vi "io_read_long_data.vi"(4 "Simulation read buffer (\"Simulation\")":string="Simulation", 6 "Block Logging (F)":bool, 8 "error in":errorcluster, 10 "Max chunk read bytes count (65536)":u32=65536, 11 "VISA resource name":refnum<visa-resource-name>) -> (0 "error out":errorcluster, 1 "return count":u32, 2 "read buffer":string, 3 "VISA resource name out":refnum<visa-resource-name>)   [LabVIEW 2014, in "rszvl_rsidr_core.lvlib"]
uses:
  rszvl_rsidr_core.lvlib
  type_Error_Codes.ctl
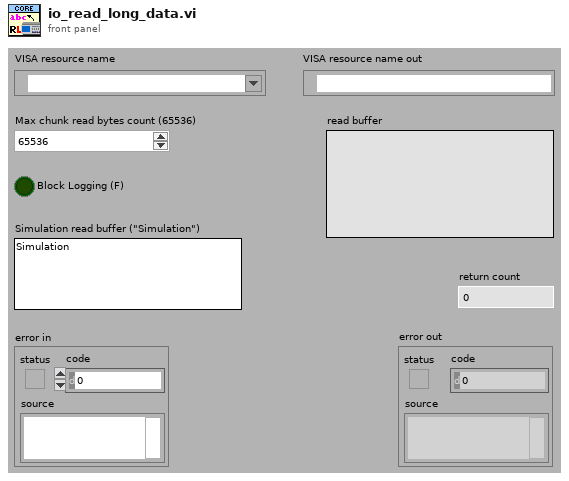
[diagram p1: front panel]
types:
  T1 = typedef "rszvl_rsidr_core.lvlib/type_Error_Codes.ctl" = enum16{"No_error", "VISA_err_ResourceNotFound", "VISA_err_Timeout", "VISA_warn_MoreDataAvailable", "RS_err_MissingCallback", "RS_err_InvalidAttribute", "RS_err_InvalidValue", "RS_err_UnknownResource", "RS_err_AlreadyInitialized", "RS_err_InstrumentStatus", "RS_err_BadRepCapName", "RS_err_TypesMismatch", "RS_err_ValueNotSupported", "RS_err_InvalidRngTable", "RS_err_IDqueryFail", "RS_err_UnexpResponse", "VISA_warn_ConfigNotLoaded", "RS_err_AttributeNotReadable", "RS_err_AttributeNotWritable", "RS_err_InstrumentType", "RS_err_InstrumentOption", "VISA_err_InvalidSize", "RS_err_ReliabilityIndicator", "VISA_warn_UnknownStatus", "VISA_warn_TermCharRead", "VISA_err_IO_error"}
  T2 = typedef "rszvl_rsidr_core.lvlib/type_Session_Data.ctl" = cluster{"Instr type":string, "Instr type for err. msg.":string, "Installed Options":string[], "OPC Timeout":i32, "Query Instrument Status":bool, "Check Range":bool, "Check Options":bool, "Add LF to Write":bool, "Simulate":bool, "Logging":bool, "Logging params":variant, "Interface Type":enum16{"Unknown", "GPIB", "VXI", "GPIB_VXI", "ASRL", "PXI", "TCPIP", "USB", "SOCKET"}, "Fast Sweep":i32, "AdditionalFlags":i32, "WaitBeforeWrite":i32, "WaitBeforeRead":i32, "BinDataChunkSize":i64}
  T3 = enum16{"Unknown", "GPIB", "VXI", "GPIB_VXI", "ASRL", "PXI", "TCPIP", "USB", "SOCKET"}
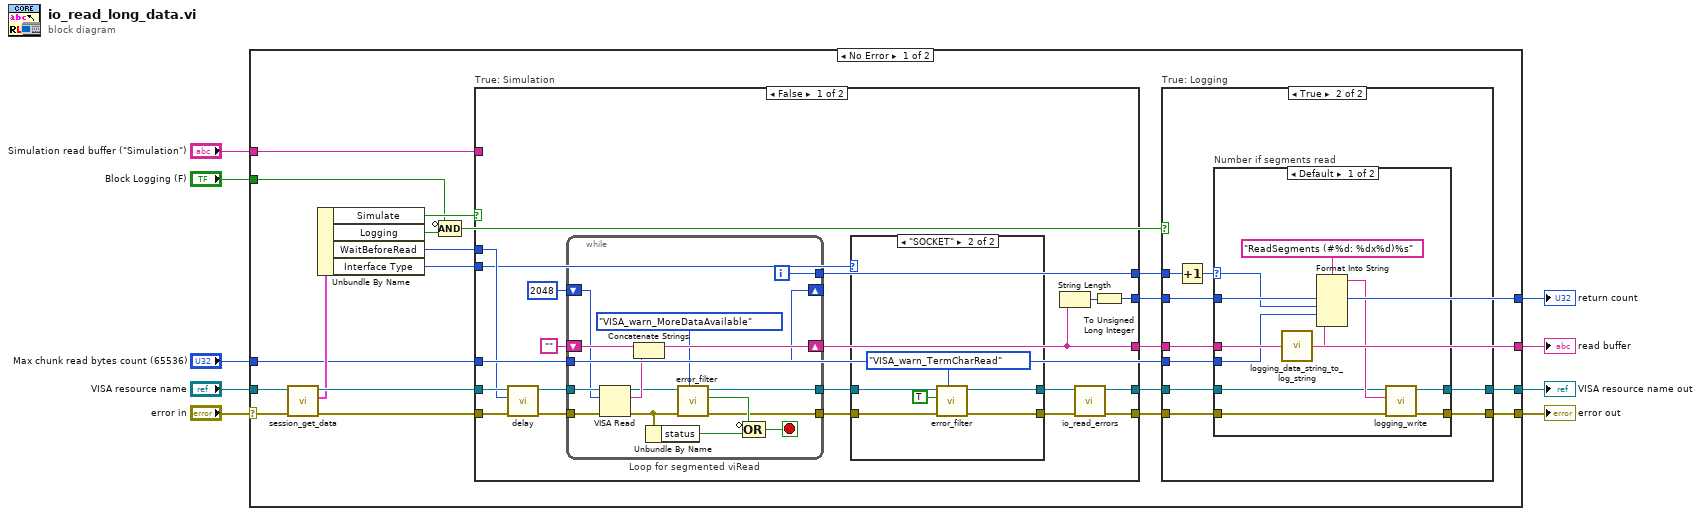
[diagram p0: block diagram]
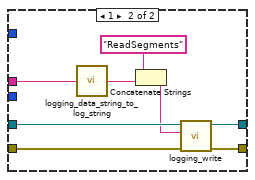
[diagram p3: hidden frame]
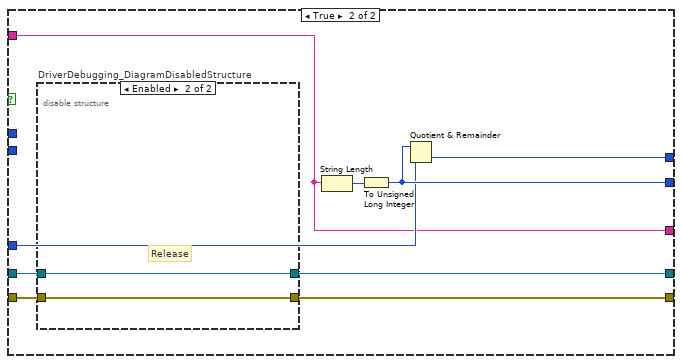
[diagram p5: hidden frame]
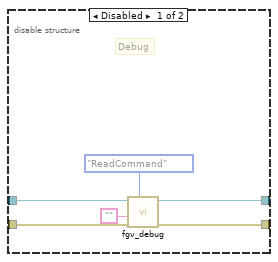
[diagram p6: hidden frame]
diagram:
  n1 = case shown="No Error" "error in" {
    selector: "error in" -> [w29 w121]
    tunnel: [w20 w121] -> w4
    tunnel: "Max chunk read bytes count (65536)" -> [w15 _]
    tunnel: [w16 _] -> w8
    tunnel: "VISA resource name" -> [w28 w120]
    tunnel: [w17 _] -> w5
    tunnel: [w19 w120] -> w3
    tunnel: "Simulation read buffer (\"Simulation\")" -> [w11 _]
    tunnel: "Block Logging (F)" -> [w10 _]
    frame No Error {
      n2 = call "session_get_data.vi"("error in"=w29, "VISA resource name"=w28) -> ("error out"=w27:errorcluster, "Session User Data out"=w25:T2, "VISA resource name out"=w26:refnum<visa-resource-name>)  [unwired: 7 in]
      n3 = Unbundle By Name(w25) -> ("Simulate"=w24:bool, "Logging"=w23:bool, "WaitBeforeRead"=w13:i32, "Interface Type"=w12:T3)
      n4 = Compound Arithmetic op=AND(invert w10, w23) -> (w14:bool)
      n5 = case "True: Simulation" shown="False" w24 {
        tunnel: [w73 w105] -> w22
        tunnel: [w76 w103] -> w16
        tunnel: [w78 w109] -> w17
        tunnel: w27 -> [w71 w107]
        tunnel: w26 -> [w70 w106]
        tunnel: [w72 w104] -> w21
        tunnel: w15 -> [w60 w108]
        tunnel: [w74 w110] -> w18
        tunnel: w13 -> [w67 _]
        tunnel: w12 -> [w64 _]
        tunnel: w11 -> [_ w103]
        frame False {
          n6 = call "delay.vi"("error in"=w71, "Milliseconds to wait"=w67, "VISA resource name"=w70) -> ("error out"=w69:errorcluster, "VISA resource name out"=w68:refnum<visa-resource-name>)  [unwired: 7 in]
          n7 = while "Loop for segmented viRead" {
            shift-left: "" ("Empty String Constant") -> [w101]
            shift-right: [w99] -> w76
            tunnel: w68 -> [w102]
            tunnel: w69 -> [w100]
            tunnel: [w92] -> w66
            tunnel: [w89] -> w63
            tunnel: [w91] -> w74
            shift-right: [w87] -> _
            shift-left: u32 2048 ("Max chunk read bytes count (65536)") -> [w88]
            tunnel: w60 -> [w87]
            i -> [w91]
            stop <- w96 stop-if-true
            n8 = VISA Read(VISA resource name=w102, byte count=w88, error in (no error)=w100) -> (VISA resource name out=w90:refnum<visa-resource-name>, read buffer=w93:string, error out=w98:errorcluster)  [unwired: 1 out]
            n9 = Concatenate Strings(w101, w93) -> (w99:string)
            n10 = Unbundle By Name(w98) -> ("status"=w97:bool)
            n11 = call "error_filter.vi"("Error Enum in"=type_Error_Codes."VISA_warn_MoreDataAvailable" ("Code to detect"), "error in"=w98, "VISA resource name"=w90) -> ("error out"=w92:errorcluster, "Code Detected"=w94:bool, "VISA resource name out"=w89:refnum<visa-resource-name>)  [unwired: 6 in]
            n12 = Compound Arithmetic op=OR(invert w94, w97) -> (w96:bool)
          }
          n13 = case shown="\"SOCKET\"" w64 {
            tunnel: w66 -> [w80 w86]
            tunnel: [w80 w84] -> w65
            tunnel: w63 -> [w79 w82]
            tunnel: [w79 w81] -> w62
            frame Default {
            }
            frame "SOCKET" {
              n14 = call "error_filter.vi"("Error Enum in"=type_Error_Codes."VISA_warn_TermCharRead" ("Code to detect"), "error in"=w86, "Clear detected code (F)"=TRUE, "VISA resource name"=w82) -> ("error out"=w84:errorcluster, "VISA resource name out"=w81:refnum<visa-resource-name>)  [unwired: 5 in, 1 out]
            }
          }
          n15 = String Length(string=w76) -> (length=w75:i32)
          n16 = call "io_read_errors.vi"("error in"=w65, "VISA resource name"=w62) -> ("error out"=w73:errorcluster, "VISA resource name out"=w72:refnum<visa-resource-name>)  [unwired: 8 in]
          n17 = To Unsigned Long Integer(number=w75) -> (unsigned 32bit integer=w78:u32)
        }
        frame True {
          n18 = disable-structure "DriverDebugging_DiagramDisabledStructure" shown="Enabled" {
            disable-tunnel: w107 -> [w116 w118]
            disable-tunnel: [w114 w118] -> w105
            disable-tunnel: w106 -> [w115 w119]
            disable-tunnel: [w113 w119] -> w104
            frame Disabled {
              # "Debug"
              n19 = call "fgv_debug.vi"("Operation"=enum16{"Reset", "ReadCommand", "SetCommand"}."ReadCommand", "error in"=w116, "Command in"="" ("Empty String Constant"), "VISA resource name"=w115) -> ("error out"=w114:errorcluster, "VISA resource name out"=w113:refnum<visa-resource-name>)  [unwired: 6 in]
            }
            frame Enabled {
              # "Release"
            }
          }
          n20 = String Length(string=w103) -> (length=w111:i32)
          n21 = To Unsigned Long Integer(number=w111) -> (unsigned 32bit integer=w109:u32)
          n22 = Quotient & Remainder(x=w109, y=w108) -> (floor(x/y)=w110:u32)  [unwired: 1 out]
        }
      }
      n23 = case "True: Logging" shown="True" w14 {
        tunnel: w21 -> [w30 w34]
        tunnel: w22 -> [w31 w35]
        tunnel: [w31 w33] -> w20
        tunnel: [w30 w32] -> w19
        tunnel: w18 -> [_ w39]
        tunnel: w16 -> [_ w40]
        tunnel: w17 -> [_ w37]
        tunnel: w15 -> [_ w36]
        frame False {
        }
        frame True {
          n24 = Increment(x=w39) -> (x+1=w38:u32)
          n25 = case "Number if segments read" shown="Default" w38 {
            selector: w38 -> [w43 _]
            tunnel: w35 -> [w49 w59]
            tunnel: w34 -> [w48 w58]
            tunnel: [w47 w57] -> w33
            tunnel: [w46 w56] -> w32
            tunnel: w40 -> [w50 w55]
            tunnel: w37 -> [w44 _]
            tunnel: w36 -> [w42 _]
            frame Default {
              n26 = call "logging_data_string_to_log_string.vi"("Raw string to log"=w50) -> ("Result log string"=w41:string)  [unwired: 4 in]
              n27 = Format Into String(format string="ReadSegments (#%d: %dx%d)%s", w44, w43, w42, w41) -> (resulting string=w51:string)  [unwired: 2 in, 1 out]
              n28 = call "logging_write.vi"("error in"=w49, "String to write"=w51, "VISA resource name"=w48) -> ("error out"=w47:errorcluster, "VISA resource name out"=w46:refnum<visa-resource-name>)  [unwired: 7 in]
            }
            frame 1 {
              n29 = call "logging_data_string_to_log_string.vi"("Raw string to log"=w55) -> ("Result log string"=w54:string)  [unwired: 4 in]
              n30 = Concatenate Strings("ReadSegments" ("format string"), w54) -> (w52:string)
              n31 = call "logging_write.vi"("error in"=w59, "String to write"=w52, "VISA resource name"=w58) -> ("error out"=w57:errorcluster, "VISA resource name out"=w56:refnum<visa-resource-name>)  [unwired: 7 in]
            }
          }
        }
      }
    }
    frame Error {
    }
  }
  "VISA resource name out" <- w3
  "error out" <- w4
  "read buffer" <- w8
  "return count" <- w5
